vi "adjust stimulus buttons.vi"(7 "Stimulus Array":T1(array[cluster]), 8 "error in (no error)":errorcluster, 9 "Edit handle":refnum<vi>, 10 "Delete handle":refnum<vi>, 11 "stimulii handle":refnum<vi>) -> (0 "error out":errorcluster)   [LabVIEW 2021]
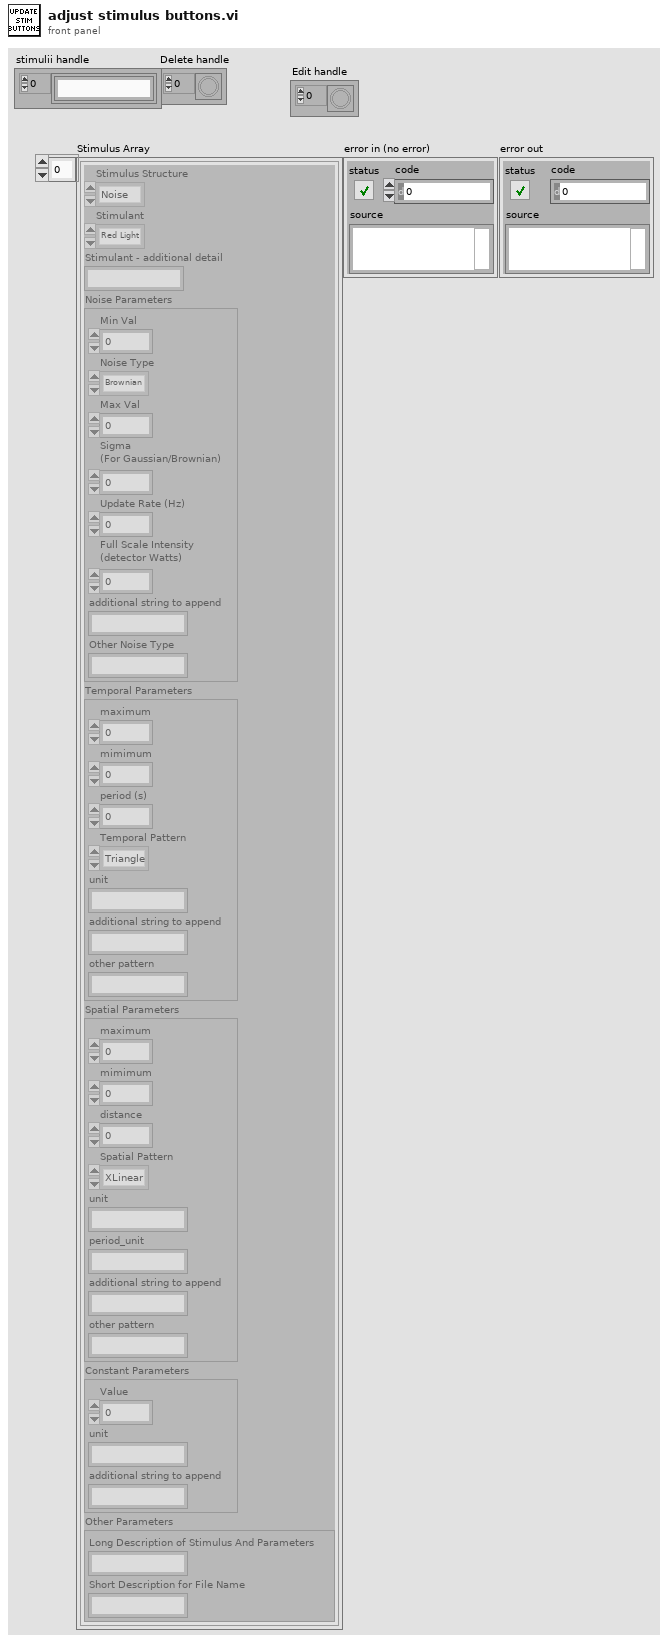
[diagram p1: front panel]
types:
  T1 = cluster{"Stimulus Structure":enum16{"Noise", "Temporal", "Spatial", "Constant", "Other"}, "Stimulant":enum16{"Red Light", "Blue Light", "Green Light", "Odor", "Temperature", "Taste", "Other"}, "Stimulant - additional detail":string, "Noise Parameters":cluster{"Min Val":dbl, "Noise Type":enum16{"Brownian", "Gaussian", "M-Sequence", "Integral of M-Sequence", "Bernoulli", "Uniform", "Other"}, "Max Val":dbl, "Sigma \n(For Gaussian/Brownian)":dbl, "Update Rate (Hz)":dbl, "Full Scale Intensity \n(detector Watts)":dbl, "additional string to append":string, "Other Noise Type":string}, "Temporal Parameters":cluster{"maximum":dbl, "mimimum":dbl, "period (s)":dbl, "Temporal Pattern":enum16{"Triangle", "Sine", "Square", "Other"}, "unit":string, "additional string to append":string, "other pattern":string}, "Spatial Parameters":cluster{"maximum":dbl, "mimimum":dbl, "distance":dbl, "Spatial Pattern":enum16{"XLinear", "YLinear", "Droplet", "Radial", "Other"}, "unit":string, "period_unit":string, "additional string to append":string, "other pattern":string}, "Constant Parameters":cluster{"Value":dbl, "unit":string, "additional string to append":string}, "Other Parameters":cluster{"Long Description of Stimulus And Parameters":string, "Short Description for File Name":string}}[]
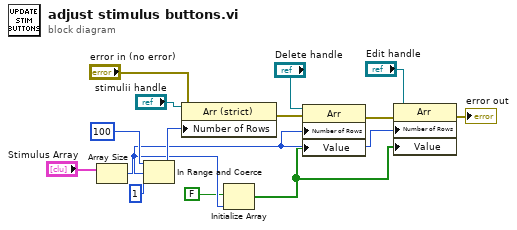
[diagram p0: block diagram]
diagram:
  n1 = Array Size(array="Stimulus Array") -> (size(s)=w3:i32)
  n2 = In Range and Coerce(upper limit=100, x=w3, lower limit=1) -> (coerced(x)=w11:i32)  [unwired: 1 out]
  n3 = property class="Arr (strict)"(reference="stimulii handle", error in="error in (no error)", "Number of Rows"=w11) -> (error out=w6:errorcluster)  [unwired: 1 out]
  n4 = Initialize Array(FALSE, w3) -> (w1:bool[])
  n5 = property class="Arr"(reference="Delete handle", error in=w6, "Number of Rows"=w3, "Value"=w1) -> (error out=w7:errorcluster)  [unwired: 1 out]
  n6 = property class="Arr"(reference="Edit handle", error in=w7, "Number of Rows"=w3, "Value"=w1) -> (error out=→"error out":errorcluster)  [unwired: 1 out]
